vi "FindTopAndBottomEdgesOld (SubVI).vi"(0 "Calibrated Image Array":T2[](array[typedef]), 1 "Fit Options":T6={"Number of Lines"=1, "Type"=enum."Best Edge Rake", "Min. Score"=10.0, "Max. Score"=1000.0, "Orientation"=0.0, "Angle Range"=45.0, "Angle Tolerance"=1.0, "Step Size"=196, "Min. SNR (db)"=0.0, "Min. Points (%)"=25.0, "Hough Iterations"=5} {"Min. Points (%)" min=0.0 max=100.0; "Min. SNR (db)" min=0.0; "Max. Score" min=0.0 max=1024.0; "Min. Score" min=0.0 max=1024.0 step=1.0}, 11 "error in (no error)":errorcluster, 12 "Templates path":path=path "C:/Users/Aerotech/Documents/BNL_ThermomechanicalStave/0_Calibration") -> (4 "Analyzed Image Array":T2[](array[typedef]), 6 "Top Edges":T5(array[cluster])=[[{"Point1 (Pixels)"={"X"=284.0, "Y"=285.3472}, "Point2 (Pixels)"={"X"=1852.0, "Y"=342.20248}, "Point1 (Real-World)"={"X"=284.0, "Y"=285.3472}, "Point2 (Real-World)"={"X"=1852.0, "Y"=342.20248}, "Angle (Pixel)"=-2.0766207872938574, "Angle (Real-World)"=-2.0766207872938574, "Score"=244.2576988070619, "Straightness"=0.07866814153400364, "Average SNR (db)"=13.758625759511817, "Calibration Valid"=TRUE}], [{"Point1 (Pixels)"={"X"=284.0, "Y"=285.33212}, "Point2 (Pixels)"={"X"=1852.0, "Y"=342.0008}, "Point1 (Real-World)"={"X"=284.0, "Y"=285.33212}, "Point2 (Real-World)"={"X"=1852.0, "Y"=342.0008}, "Angle (Pixel)"=-2.0698111412213156, "Angle (Real-World)"=-2.0698111412213156, "Score"=242.57703294941024, "Straightness"=0.11529837461588602, "Average SNR (db)"=12.63726725279762, "Calibration Valid"=TRUE}], [{"Point1 (Pixels)"={"X"=288.0, "Y"=284.97113}, "Point2 (Pixels)"={"X"=1856.0, "Y"=342.4715}, "Point1 (Real-World)"={"X"=288.0, "Y"=284.97113}, "Point2 (Real-World)"={"X"=1856.0, "Y"=342.4715}, "Angle (Pixel)"=-2.1001609084437023, "Angle (Real-World)"=-2.1001609084437023, "Score"=240.89635213216147, "Straightness"=0.06827464097552538, "Average SNR (db)"=12.705183064283393, "Calibration Valid"=TRUE}], [{"Point1 (Pixels)"={"X"=153.0, "Y"=410.42282}, "Point2 (Pixels)"={"X"=1721.0, "Y"=431.67874}, "Point1 (Real-World)"={"X"=153.0, "Y"=410.42282}, "Point2 (Real-World)"={"X"=1721.0, "Y"=431.67874}, "Angle (Pixel)"=-0.776658221860711, "Angle (Real-World)"=-0.776658221860711, "Score"=260.5042102290135, "Straightness"=0.10945376347882856, "Average SNR (db)"=13.85395164330424, "Calibration Valid"=TRUE}], [{"Point1 (Pixels)"={"X"=154.0, "Y"=410.6867}, "Point2 (Pixels)"={"X"=1722.0, "Y"=431.18222}, "Point1 (Real-World)"={"X"=154.0, "Y"=410.6867}, "Point2 (Real-World)"={"X"=1722.0, "Y"=431.18222}, "Angle (Pixel)"=-0.7488769386896038, "Angle (Real-World)"=-0.7488769386896038, "Score"=261.62465413411456, "Straightness"=0.0825086511825605, "Average SNR (db)"=13.9277311023817, "Calibration Valid"=TRUE}], [{"Point1 (Pixels)"={"X"=153.0, "Y"=410.68866}, "Point2 (Pixels)"={"X"=1721.0, "Y"=431.17807}, "Point1 (Real-World)"={"X"=153.0, "Y"=410.68866}, "Point2 (Real-World)"={"X"=1721.0, "Y"=431.17807}, "Angle (Pixel)"=-0.7486536639939473, "Angle (Real-World)"=-0.7486536639939473, "Score"=264.42577885646443, "Straightness"=0.08504378768918679, "Average SNR (db)"=14.214596716329881, "Calibration Valid"=TRUE}], [{"Point1 (Pixels)"={"X"=170.0, "Y"=441.4789}, "Point2 (Pixels)"={"X"=1738.0, "Y"=446.1428}, "Point1 (Real-World)"={"X"=170.0, "Y"=441.4789}, "Point2 (Real-World)"={"X"=1738.0, "Y"=446.1428}, "Angle (Pixel)"=-0.1704212404082558, "Angle (Real-World)"=-0.1704212404082558, "Score"=183.7535035376455, "Straightness"=0.2684447490123475, "Average SNR (db)"=14.709590108072733, "Calibration Valid"=TRUE}], [{"Point1 (Pixels)"={"X"=190.0, "Y"=441.2455}, "Point2 (Pixels)"={"X"=1758.0, "Y"=445.48163}, "Point1 (Real-World)"={"X"=190.0, "Y"=441.2455}, "Point2 (Real-World)"={"X"=1758.0, "Y"=445.48163}, "Angle (Pixel)"=-0.15479114326159896, "Angle (Real-World)"=-0.15479114326159896, "Score"=180.3921568627451, "Straightness"=0.19882038748807523, "Average SNR (db)"=13.94876466007177, "Calibration Valid"=TRUE}], [{"Point1 (Pixels)"={"X"=185.0, "Y"=441.11078}, "Point2 (Pixels)"={"X"=1753.0, "Y"=445.67474}, "Point1 (Real-World)"={"X"=185.0, "Y"=441.11078}, "Point2 (Real-World)"={"X"=1753.0, "Y"=445.67474}, "Angle (Pixel)"=-0.1667697559923643, "Angle (Real-World)"=-0.1667697559923643, "Score"=182.63305963254442, "Straightness"=0.18692307526997337, "Average SNR (db)"=14.497469805413253, "Calibration Valid"=TRUE}], [{"Point1 (Pixels)"={"X"=407.0, "Y"=454.844}, "Point2 (Pixels)"={"X"=1975.0, "Y"=469.98376}, "Point1 (Real-World)"={"X"=407.0, "Y"=454.844}, "Point2 (Real-World)"={"X"=1975.0, "Y"=469.98376}, "Angle (Pixel)"=-0.5532005609100381, "Angle (Real-World)"=-0.5532005609100381, "Score"=203.92156862745097, "Straightness"=0.09033156432138925, "Average SNR (db)"=16.237674173273582, "Calibration Valid"=TRUE}], [{"Point1 (Pixels)"={"X"=407.0, "Y"=454.735}, "Point2 (Pixels)"={"X"=1975.0, "Y"=469.81674}, "Point1 (Real-World)"={"X"=407.0, "Y"=454.735}, "Point2 (Real-World)"={"X"=1975.0, "Y"=469.81674}, "Angle (Pixel)"=-0.5510809046359758, "Angle (Real-World)"=-0.5510809046359758, "Score"=205.0420125325521, "Straightness"=0.07144511590294857, "Average SNR (db)"=14.644864859451086, "Calibration Valid"=TRUE}], [{"Point1 (Pixels)"={"X"=407.0, "Y"=454.22052}, "Point2 (Pixels)"={"X"=1975.0, "Y"=469.77655}, "Point1 (Real-World)"={"X"=407.0, "Y"=454.22052}, "Point2 (Real-World)"={"X"=1975.0, "Y"=469.77655}, "Angle (Pixel)"=-0.5684092576992881, "Angle (Real-World)"=-0.5684092576992881, "Score"=203.92156862745097, "Straightness"=0.1412673039990816, "Average SNR (db)"=15.91514851048057, "Calibration Valid"=TRUE}]], 8 "Bottom Edges":T5(array[cluster])=[[{"Point1 (Pixels)"={"X"=204.0, "Y"=1575.3654}, "Point2 (Pixels)"={"X"=1772.0, "Y"=1627.383}, "Point1 (Real-World)"={"X"=204.0, "Y"=1575.3654}, "Point2 (Real-World)"={"X"=1772.0, "Y"=1627.383}, "Angle (Pixel)"=-1.9000626776283849, "Angle (Real-World)"=-1.9000626776283849, "Score"=163.02521649528953, "Straightness"=0.4507744451365954, "Average SNR (db)"=12.848425611197095, "Calibration Valid"=TRUE}], [{"Point1 (Pixels)"={"X"=206.0, "Y"=1570.0475}, "Point2 (Pixels)"={"X"=1774.0, "Y"=1629.0887}, "Point1 (Real-World)"={"X"=206.0, "Y"=1570.0475}, "Point2 (Real-World)"={"X"=1774.0, "Y"=1629.0887}, "Angle (Pixel)"=-2.1563951033080153, "Angle (Real-World)"=-2.1563951033080153, "Score"=154.6218423282399, "Straightness"=0.8425670124335514, "Average SNR (db)"=13.086057242764024, "Calibration Valid"=TRUE}], [{"Point1 (Pixels)"={"X"=205.0, "Y"=1570.5215}, "Point2 (Pixels)"={"X"=1773.0, "Y"=1629.1553}, "Point1 (Real-World)"={"X"=205.0, "Y"=1570.5215}, "Point2 (Real-World)"={"X"=1773.0, "Y"=1629.1553}, "Angle (Pixel)"=-2.1415197113170206, "Angle (Real-World)"=-2.1415197113170206, "Score"=156.30252314548866, "Straightness"=0.6322513813515124, "Average SNR (db)"=13.03766809720698, "Calibration Valid"=TRUE}], [{"Point1 (Pixels)"={"X"=325.0, "Y"=1696.2217}, "Point2 (Pixels)"={"X"=1893.0, "Y"=1713.9342}, "Point1 (Real-World)"={"X"=325.0, "Y"=1696.2217}, "Point2 (Real-World)"={"X"=1893.0, "Y"=1713.9342}, "Angle (Pixel)"=-0.6471987274858038, "Angle (Real-World)"=-0.6471987274858038, "Score"=243.13725490196077, "Straightness"=0.15845546024406645, "Average SNR (db)"=17.086258204590646, "Calibration Valid"=TRUE}], [{"Point1 (Pixels)"={"X"=333.0, "Y"=1695.9786}, "Point2 (Pixels)"={"X"=1901.0, "Y"=1714.3751}, "Point1 (Real-World)"={"X"=333.0, "Y"=1695.9786}, "Point2 (Real-World)"={"X"=1901.0, "Y"=1714.3751}, "Angle (Pixel)"=-0.6721889611182643, "Angle (Real-World)"=-0.6721889611182643, "Score"=244.2576988070619, "Straightness"=0.15332228619744986, "Average SNR (db)"=16.84450305026053, "Calibration Valid"=TRUE}], [{"Point1 (Pixels)"={"X"=333.0, "Y"=1696.4978}, "Point2 (Pixels)"={"X"=1901.0, "Y"=1713.8031}, "Point1 (Real-World)"={"X"=333.0, "Y"=1696.4978}, "Point2 (Real-World)"={"X"=1901.0, "Y"=1713.8031}, "Angle (Pixel)"=-0.6323181983453772, "Angle (Real-World)"=-0.6323181983453772, "Score"=245.3781576717601, "Straightness"=0.1831879021447923, "Average SNR (db)"=17.244463055985563, "Calibration Valid"=TRUE}], [{"Point1 (Pixels)"={"X"=892.0, "Y"=1262.0977}, "Point2 (Pixels)"={"X"=2460.0, "Y"=1308.8115}, "Point1 (Real-World)"={"X"=892.0, "Y"=1262.0977}, "Point2 (Real-World)"={"X"=2460.0, "Y"=1308.8115}, "Angle (Pixel)"=-1.706451530017727, "Angle (Real-World)"=-1.706451530017727, "Score"=21.848740297205307, "Straightness"=8.045014544831348, "Average SNR (db)"=5.552365578076705, "Calibration Valid"=TRUE}], [{"Point1 (Pixels)"={"X"=892.0, "Y"=1276.9999}, "Point2 (Pixels)"={"X"=2460.0, "Y"=1292.2001}, "Point1 (Real-World)"={"X"=892.0, "Y"=1276.9999}, "Point2 (Real-World)"={"X"=2460.0, "Y"=1292.2001}, "Angle (Pixel)"=-0.5554080101657966, "Angle (Real-World)"=-0.5554080101657966, "Score"=39.77591196695963, "Straightness"=2.053305015267911, "Average SNR (db)"=6.0777660374169304, "Calibration Valid"=TRUE}], [{"Point1 (Pixels)"={"X"=0.0, "Y"=0.0}, "Point2 (Pixels)"={"X"=0.0, "Y"=0.0}, "Point1 (Real-World)"={"X"=0.0, "Y"=0.0}, "Point2 (Real-World)"={"X"=0.0, "Y"=0.0}, "Angle (Pixel)"=0.0, "Angle (Real-World)"=0.0, "Score"=0.0, "Straightness"=0.0, "Average SNR (db)"=0.0, "Calibration Valid"=FALSE}], [{"Point1 (Pixels)"={"X"=-0.0, "Y"=1736.858}, "Point2 (Pixels)"={"X"=1568.0, "Y"=1752.6415}, "Point1 (Real-World)"={"X"=-0.0, "Y"=1736.858}, "Point2 (Real-World)"={"X"=1568.0, "Y"=1752.6415}, "Angle (Pixel)"=-0.5767197079329028, "Angle (Real-World)"=-0.5767197079329028, "Score"=145.09803921568627, "Straightness"=0.1480317125847858, "Average SNR (db)"=13.230952595144498, "Calibration Valid"=TRUE}], [{"Point1 (Pixels)"={"X"=1.0, "Y"=1736.8511}, "Point2 (Pixels)"={"X"=1569.0, "Y"=1752.5498}, "Point1 (Real-World)"={"X"=1.0, "Y"=1736.8511}, "Point2 (Real-World)"={"X"=1569.0, "Y"=1752.5498}, "Angle (Pixel)"=-0.5736255680578705, "Angle (Real-World)"=-0.5736255680578705, "Score"=143.97759531058517, "Straightness"=0.14210673230497195, "Average SNR (db)"=12.691481631077137, "Calibration Valid"=TRUE}], [{"Point1 (Pixels)"={"X"=-0.0, "Y"=1736.7153}, "Point2 (Pixels)"={"X"=1568.0, "Y"=1751.6721}, "Point1 (Real-World)"={"X"=-0.0, "Y"=1736.7153}, "Point2 (Real-World)"={"X"=1568.0, "Y"=1751.6721}, "Angle (Pixel)"=-0.5465153360610442, "Angle (Real-World)"=-0.5465153360610442, "Score"=143.4173733580346, "Straightness"=0.16803427059093384, "Average SNR (db)"=12.70203491370303, "Calibration Valid"=TRUE}]], 10 "Array of Edge Endpoint Arrays":sgl[][][](array[numeric])=[[[284.0, 285.3472, 0.0], [1852.0, 342.20248, 0.0], [204.0, 1575.3654, 0.0], [1772.0, 1627.383, 0.0]], [[284.0, 285.33212, 0.0], [1852.0, 342.0008, 0.0], [206.0, 1570.0475, 0.0], [1774.0, 1629.0887, 0.0]], [[288.0, 284.97113, 0.0], [1856.0, 342.4715, 0.0], [205.0, 1570.5215, 0.0], [1773.0, 1629.1553, 0.0]], [[153.0, 410.42282, 0.0], [1721.0, 431.67874, 0.0], [325.0, 1696.2217, 0.0], [1893.0, 1713.9342, 0.0]], [[154.0, 410.6867, 0.0], [1722.0, 431.18222, 0.0], [333.0, 1695.9786, 0.0], [1901.0, 1714.3751, 0.0]], [[153.0, 410.68866, 0.0], [1721.0, 431.17807, 0.0], [333.0, 1696.4978, 0.0], [1901.0, 1713.8031, 0.0]], [[170.0, 441.4789, 0.0], [1738.0, 446.1428, 0.0], [892.0, 1262.0977, 0.0], [2460.0, 1308.8115, 0.0]], [[190.0, 441.2455, 0.0], [1758.0, 445.48163, 0.0], [892.0, 1276.9999, 0.0], [2460.0, 1292.2001, 0.0]], [[185.0, 441.11078, 0.0], [1753.0, 445.67474, 0.0], [0.0, 0.0, 0.0], [0.0, 0.0, 0.0]], [[407.0, 454.844, 0.0], [1975.0, 469.98376, 0.0], [-0.0, 1736.858, 0.0], [1568.0, 1752.6415, 0.0]], [[407.0, 454.735, 0.0], [1975.0, 469.81674, 0.0], [1.0, 1736.8511, 0.0], [1569.0, 1752.5498, 0.0]], [[407.0, 454.22052, 0.0], [1975.0, 469.77655, 0.0], [-0.0, 1736.7153, 0.0], [1568.0, 1751.6721, 0.0]]], 15 "error in (no error) 2":errorcluster)   [LabVIEW 2016]
uses:
  <vilib>/vision/Measure.llb/Straight Edge Options.ctl
  <vilib>/vision/Measure.llb/Straight Edge Process.ctl
  <vilib>/vision/Image Controls.llb/IMAQ Image.ctl
panel:
  out "Matches (pixel) Bottom":T1(array[cluster])
  out "Matches (pixel)":T1(array[cluster])
  out "Images Array":T2[](array[plugin-control])=["image_0_-670_-89_-3", "image_1_-670_-89_-3", "image_2_-670_-89_-3", "image_3_-670_-89_-3", "image_4_-670_-89_-3", "image_5_-390_-89_-3", "image_6_-390_-89_-3", "image_7_-390_-89_-3", "image_8_-390_-89_-3", "image_9_-390_-89_-3", "image_10_-96_-89_-3", "image_11_-96_-89_-3", "image_12_-96_-89_-3", "image_13_-96_-89_-3", "image_14_-96_-89_-3", "image_15_198_-89_-3", "image_16_198_-89_-3", "image_17_198_-89_-3", "image_18_198_-89_-3", "image_19_198_-89_-3", "image_20_492_-89_-3", "image_21_492_-89_-3", "image_22_492_-89_-3", "image_23_492_-89_-3", "image_24_492_-89_-3"]
  out "Filenames Array":string[](array[string])
  in  "Naming Convention":string="image_442_-22_00.png"
  in  "Images Directory":path=path "C:/Users/sciollalab/Desktop/dots1-12-16-2016/dots_-146,-22"
  out "Template Image 2":T2
  in  "Search Rect":T3={"Left"=0, "Top"=0, "Right"=2147483647, "Bottom"=2147483647, "Rotation"=0.0} {"Rotation" format="%.2f"; "Left" scale=0.0..1024.0; "Right" scale=0.0..1024.0}
  in  "Pattern Match Settings":T4={"Algorithm"=2, "Number of Matches Requested"=1, "Minimum Match Score"=700.0, "SubPixel Accuracy"=TRUE, "Rotation Angle Ranges"=[{"Start"=-90.0, "End"=90.0}], "Show Search Area"=FALSE, "Show Result"=TRUE} {"Rotation Angle Ranges"."End" format="%.1f"; "Rotation Angle Ranges"."Start" format="%.1f"; "Minimum Match Score" min=0 max=1000 format="%.2f"; "Number of Matches Requested" min=1; "Algorithm" items=["All", "Low Discrepancy Sampling", "Grayscale Value Pyramid", "Gradients Pyramid"]}
  out "Template Image":T2
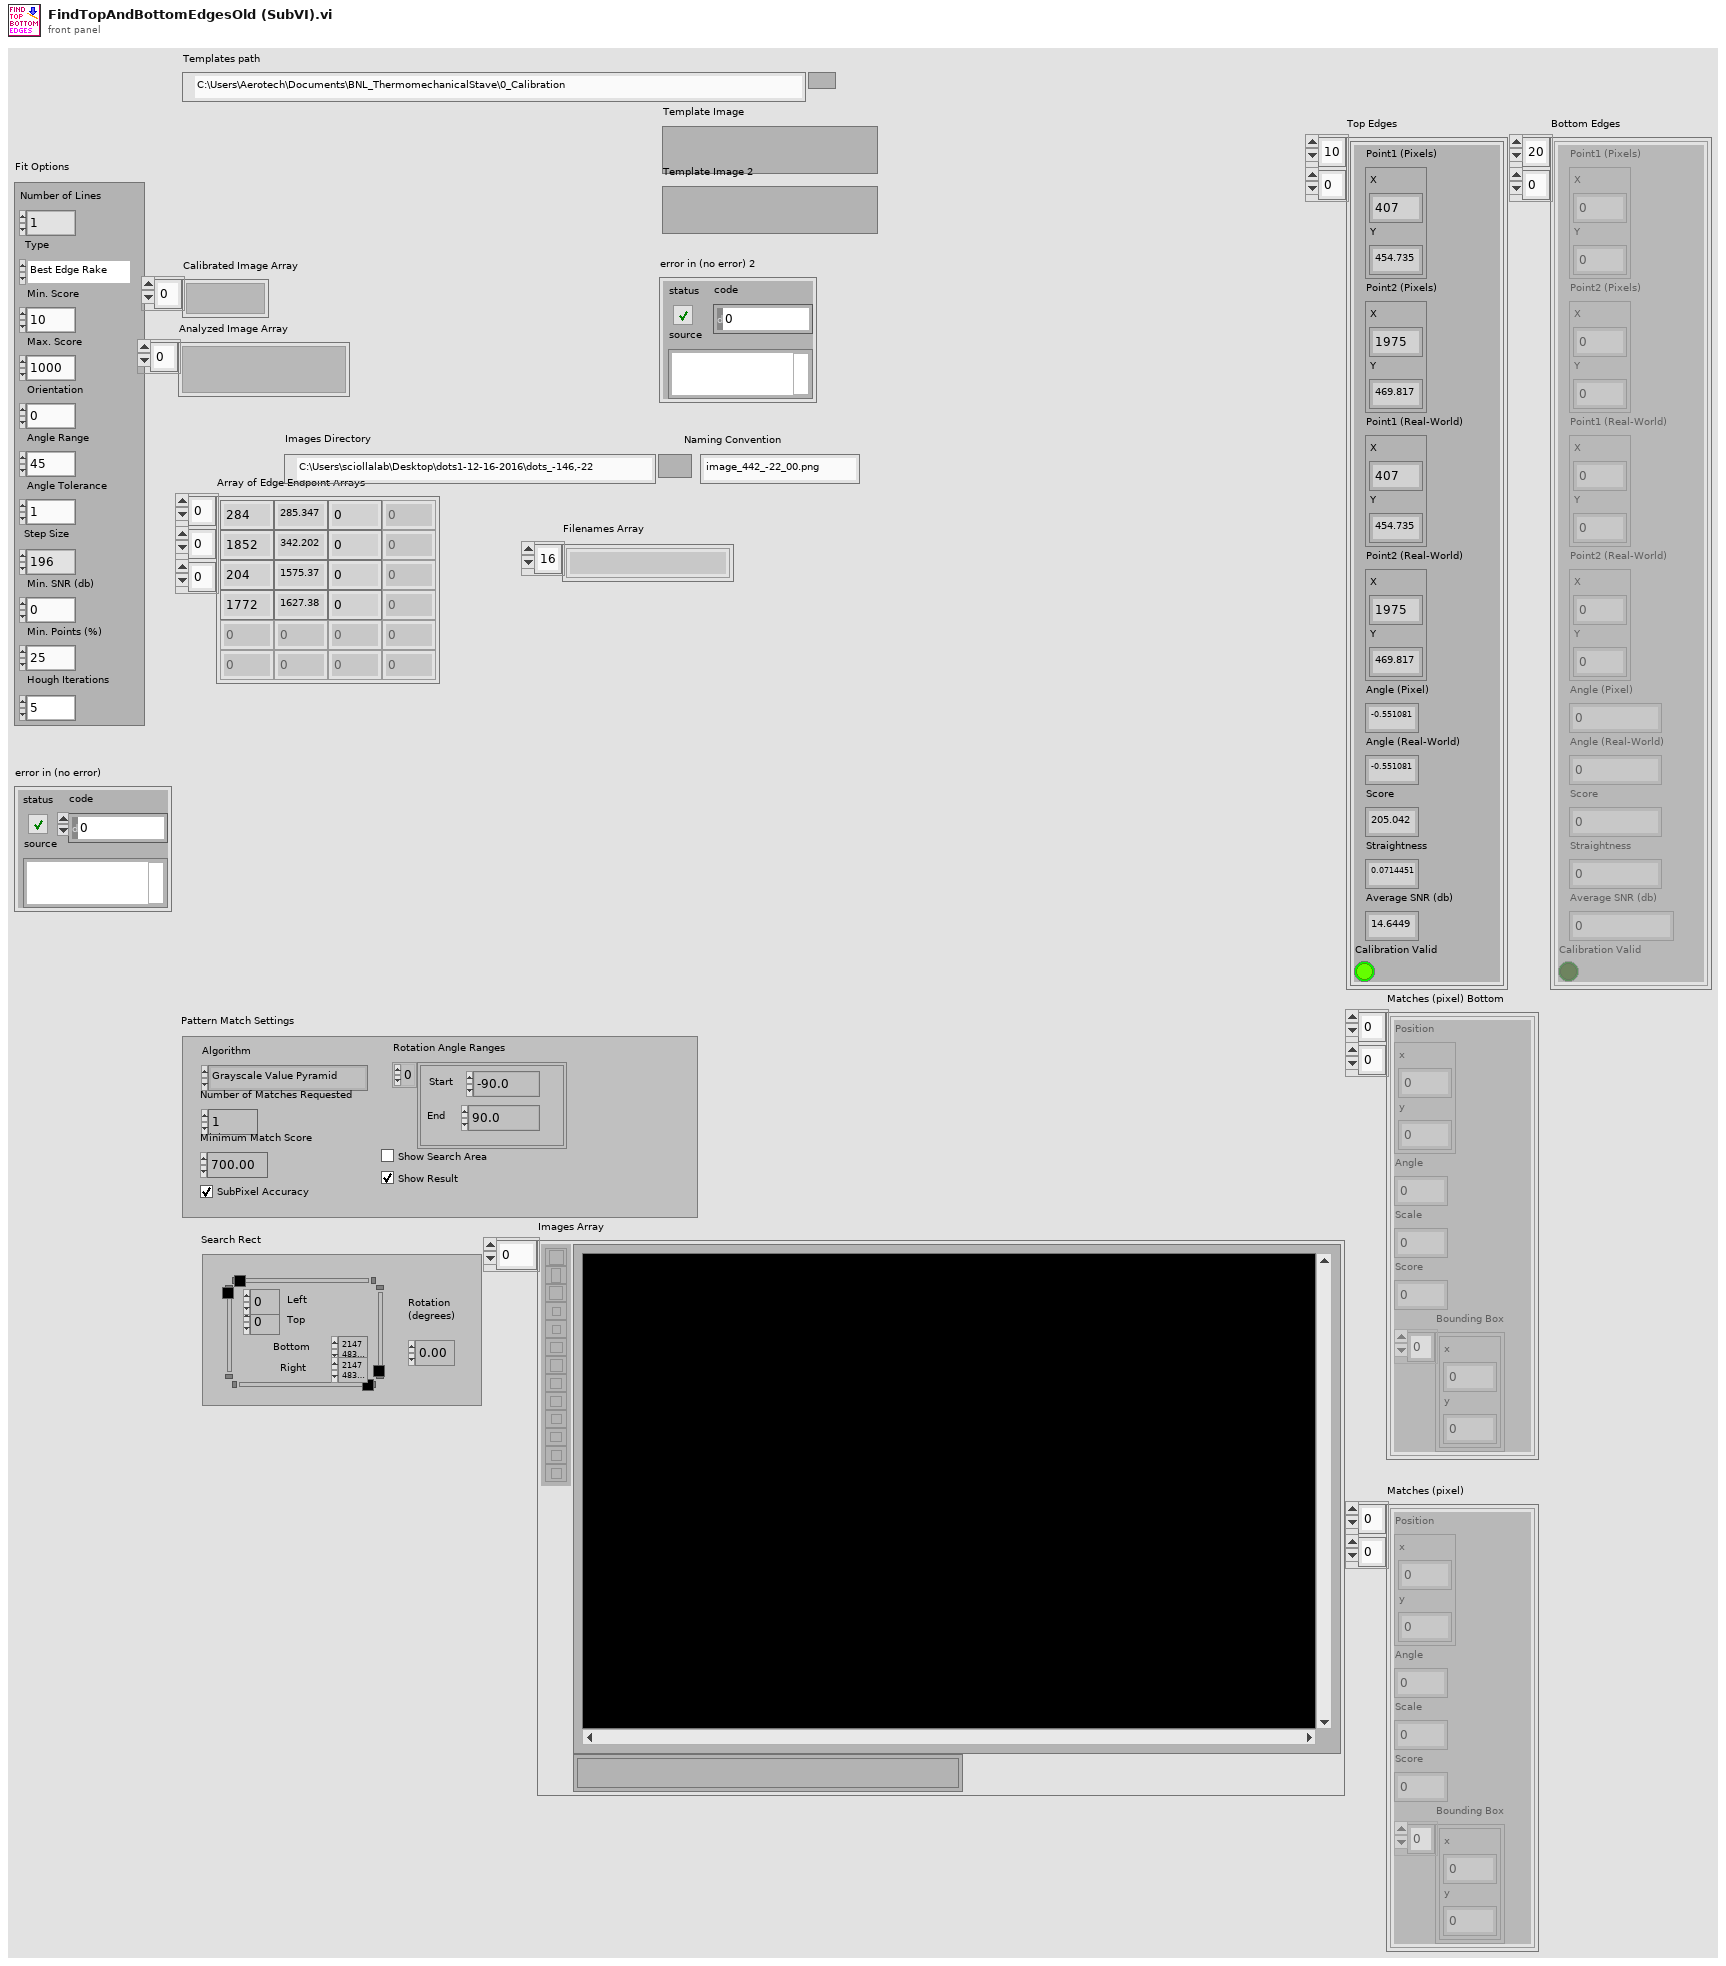
[diagram p1: front panel]
types:
  T1 = cluster{"Position":cluster{"x":sgl, "y":sgl}, "Angle":sgl, "Scale":sgl, "Score":sgl, "Bounding Box":cluster{"x":sgl, "y":sgl}[]}[][]
  T2 = typedef "IMAQ Image.ctl" = refnum<image>
  T3 = typedef "IMAQ Rectangle" = cluster{"Left":i32, "Top":i32, "Right":i32, "Bottom":i32, "Rotation":dbl}
  T4 = cluster{"Algorithm":i32, "Number of Matches Requested":i32, "Minimum Match Score":sgl, "SubPixel Accuracy":bool, "Rotation Angle Ranges":cluster{"Start":sgl, "End":sgl}[], "Show Search Area":bool, "Show Result":bool}
  T5 = cluster{"Point1 (Pixels)":cluster{"X":sgl, "Y":sgl}, "Point2 (Pixels)":cluster{"X":sgl, "Y":sgl}, "Point1 (Real-World)":cluster{"X":sgl, "Y":sgl}, "Point2 (Real-World)":cluster{"X":sgl, "Y":sgl}, "Angle (Pixel)":dbl, "Angle (Real-World)":dbl, "Score":dbl, "Straightness":dbl, "Average SNR (db)":dbl, "Calibration Valid":bool}[][]
  T6 = typedef "Straight Edge Options.ctl" = cluster{"Number of Lines":i32, "Type":T7, "Min. Score":dbl, "Max. Score":dbl, "Orientation":dbl, "Angle Range":dbl, "Angle Tolerance":dbl, "Step Size":u32, "Min. SNR (db)":dbl, "Min. Points (%)":dbl, "Hough Iterations":i32}
  T7 = typedef "Straight Edge Process.ctl" = enum32{"First Edge Rake", "Best Edge Rake", "Hough Edge Rake", "First Edge Projection", "Best Edge Projection"}
  T8 = cluster{"Point1 (Pixels)":cluster{"X":sgl, "Y":sgl}, "Point2 (Pixels)":cluster{"X":sgl, "Y":sgl}, "Point1 (Real-World)":cluster{"X":sgl, "Y":sgl}, "Point2 (Real-World)":cluster{"X":sgl, "Y":sgl}, "Angle (Pixel)":dbl, "Angle (Real-World)":dbl, "Score":dbl, "Straightness":dbl, "Average SNR (db)":dbl, "Calibration Valid":bool}[]
  T9 = cluster{"Point1 (Pixels)":cluster{"X":sgl, "Y":sgl}, "Point2 (Pixels)":cluster{"X":sgl, "Y":sgl}, "Point1 (Real-World)":cluster{"X":sgl, "Y":sgl}, "Point2 (Real-World)":cluster{"X":sgl, "Y":sgl}, "Angle (Pixel)":dbl, "Angle (Real-World)":dbl, "Score":dbl, "Straightness":dbl, "Average SNR (db)":dbl, "Calibration Valid":bool}
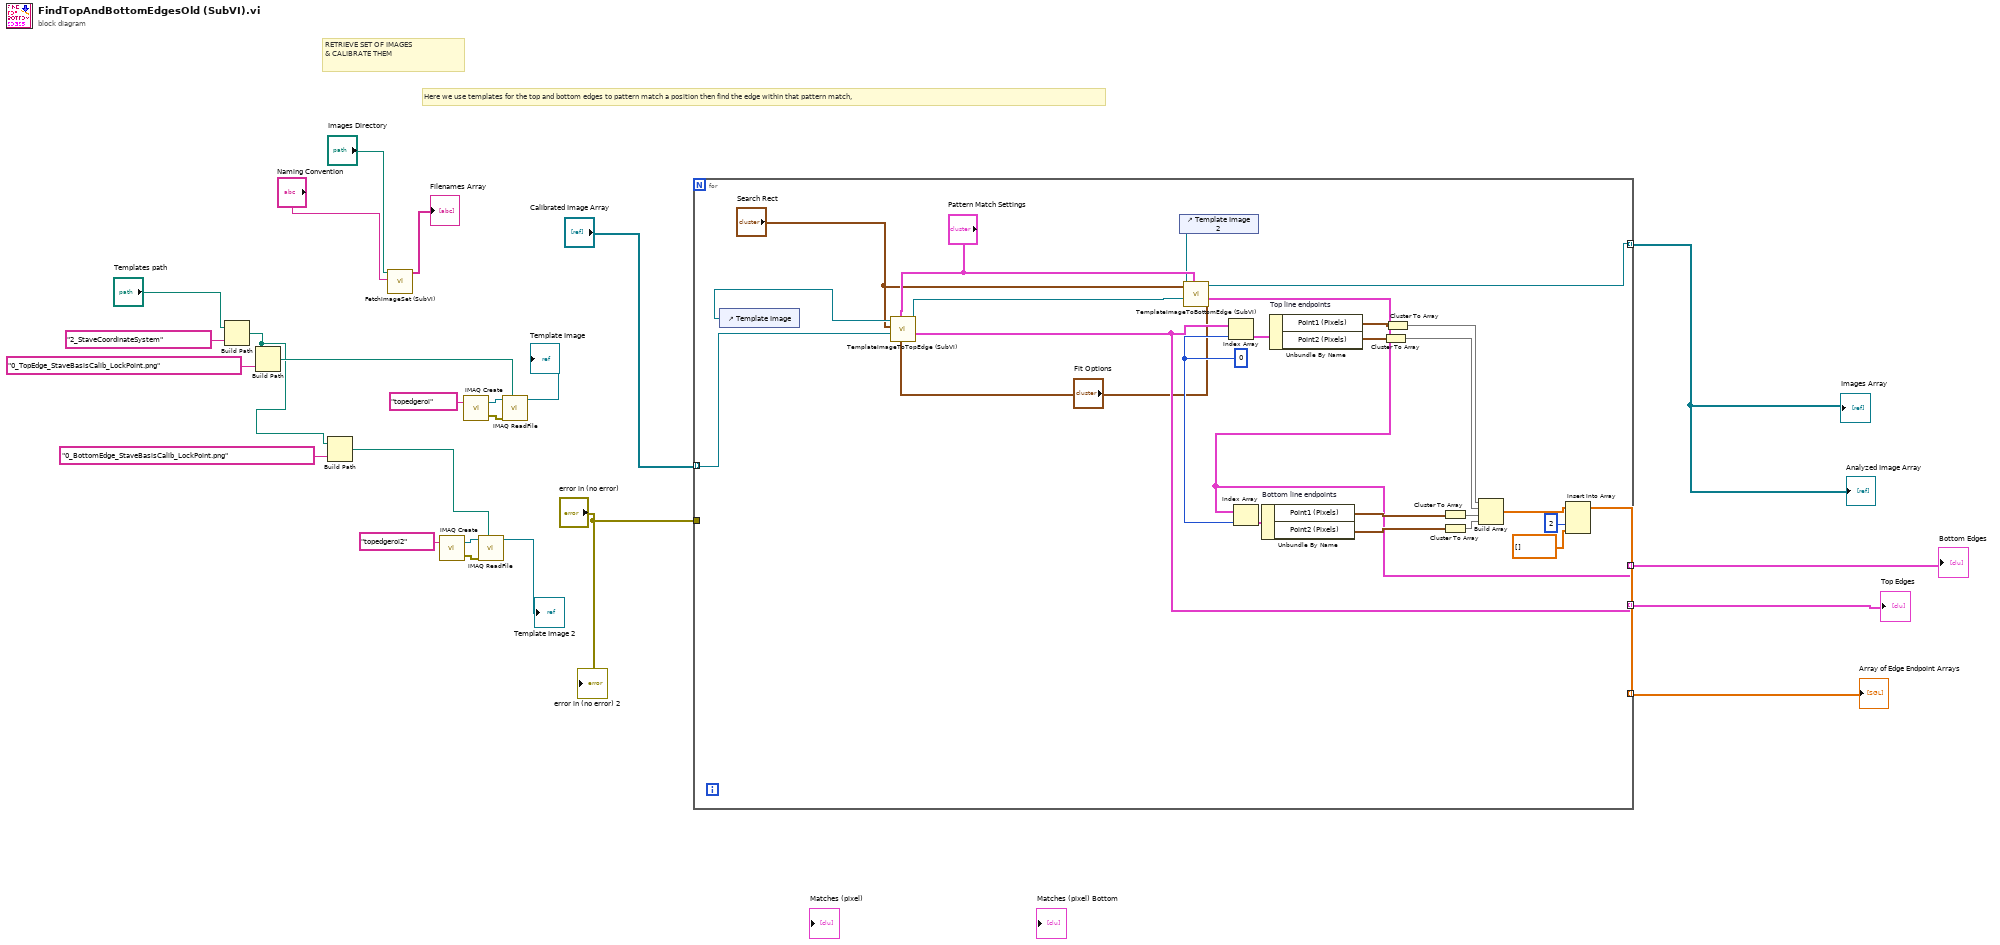
[diagram p0: block diagram]
diagram:
  # "RETRIEVE SET OF IMAGES\n& CALIBRATE THEM"
  # "Here we use templates for the top and bottom edges to pattern match a position then find the edge within that pattern match,"
  n1 = Build Path(base path="Templates path", name or relative path="2_StaveCoordinateSystem") -> (appended path=w6:path)
  n2 = Build Path(base path=w6, name or relative path="0_TopEdge_StaveBasisCalib_LockPoint.png") -> (appended path=w7:path)
  n3 = Build Path(base path=w6, name or relative path="0_BottomEdge_StaveBasisCalib_LockPoint.png") -> (appended path=w9:path)
  n4 = call "FetchImageSet (SubVI).vi"("Naming Convention"="Naming Convention", "Images Directory"="Images Directory") -> ("Filenames Array"=→"Filenames Array":string[])  [unwired: 7 in, 2 out]
  n5 = call "IMAQ Create"("Image Name"="topedgeroi2") -> ("New Image"=w15:T2, "error out"=w16:errorcluster)  [unwired: 4 in]
  n6 = call "IMAQ Create"("Image Name"="topedgeroi") -> ("New Image"=w19:T2, "error out"=w20:errorcluster)  [unwired: 4 in]
  n7 = call "IMAQ ReadFile"("File Path"=w9, "error in (no error)"=w16, "Image"=w15) -> ("Image Out"=→"Template Image 2":T2)  [unwired: 4 in, 4 out]
  n8 = call "IMAQ ReadFile"("File Path"=w7, "error in (no error)"=w20, "Image"=w19) -> ("Image Out"=→"Template Image":T2)  [unwired: 4 in, 4 out]
  n9 = for {
    tunnel: "Calibrated Image Array" -> [w34] mode=indexing
    tunnel: "error in (no error)" -> [_]
    tunnel: [w25] -> w2 mode=indexing
    tunnel: [w29] -> w24 mode=indexing
    tunnel: [w27] -> w23 mode=indexing
    tunnel: [w35] -> w22 mode=indexing
    w49 = 0 ("index")
    n10 = control-ref of="Template Image"() -> (w31:refnum<vi>)
    n11 = call "TemplateImageToTopEdge (SubVI).vi"("Line Fit Options"="Fit Options", "Pattern Match Settings"="Pattern Match Settings", "Calibrated Image"=w34, "Search Rect"="Search Rect", "GenClassTagFlatRef in"=w31) -> ("Straight Edges"=w29:T8, "Refnum out"=w28:T2)  [unwired: 3 in, 2 out]
    n12 = control-ref of="Template Image 2"() -> (w32:refnum<vi>)
    n13 = call "TemplateImageToBottomEdge (SubVI).vi"("Line Fit Options"="Fit Options", "Pattern Match Settings"="Pattern Match Settings", "Calibrated Image"=w28, "Search Rect"="Search Rect", "GenClassTagFlatRef in"=w32) -> ("Straight Edges"=w27:T8, "Refnum out"=w25:T2)  [unwired: 4 in, 1 out]
    n14 = Index Array(array=w29, index=w49) -> (element=w48:T9)
    n15 = Index Array(array=w27, index=w49) -> (element=w47:T9)
    n16 = Unbundle By Name "Bottom line endpoints"(w47) -> ("Point1 (Pixels)"=w38:cluster{"X":sgl, "Y":sgl}, "Point2 (Pixels)"=w39:cluster{"X":sgl, "Y":sgl})
    n17 = Unbundle By Name "Top line endpoints"(w48) -> ("Point1 (Pixels)"=w46:cluster{"X":sgl, "Y":sgl}, "Point2 (Pixels)"=w45:cluster{"X":sgl, "Y":sgl})
    n18 = Cluster To Array(cluster=w45) -> (array=w43:sgl[])
    n19 = Cluster To Array(cluster=w46) -> (array=w44:sgl[])
    n20 = Cluster To Array(cluster=w38) -> (array=w37:sgl[])
    n21 = Cluster To Array(cluster=w39) -> (array=w36:sgl[])
    n22 = Build Array(w44, w43, w37, w36) -> (w42:sgl[][])
    n23 = Insert Into Array(array=w42, index (col)=2 ("disabled index (col)"), new element=sgl[] [] ("new element/subarray")) -> (w35:sgl[][])  [unwired: 1 in]
  }
  "Analyzed Image Array" <- w2
  "Top Edges" <- w24
  "Bottom Edges" <- w23
  "Array of Edge Endpoint Arrays" <- w22
  "Images Array" <- w2
  "error in (no error) 2" <- "error in (no error)"
